vi "PhotonMultiTargetPNPResult_unpack.vi"(9 "StartByte":i32, 11 "RawData":u8[](array[numeric])) -> (1 "NextByte":i32, 3 "MultiTargetPNP_Result":T1={"PhotonPNPResult"={"IsPresent"=FALSE, "bestReprojErr"=0.0, "altReprojErr"=0.0, "ambiguity"=0.0, "Best"={"TRANSLATION3D"={"X"=0.0, "Y"=0.0, "Z"=0.0}, "ROTATION3D"={"Q_quaternion"={"R"=1.0, "V"=[0.0, 0.0, 0.0]}}, "XF"=FALSE}, "Alt"={"TRANSLATION3D"={"X"=0.0, "Y"=0.0, "Z"=0.0}, "ROTATION3D"={"Q_quaternion"={"R"=1.0, "V"=[0.0, 0.0, 0.0]}}, "XF"=FALSE}}, "FiducialIDsUsed"=[]} {"PhotonPNPResult"."Alt"."TRANSLATION3D"."Z" format="%14.3f"; "PhotonPNPResult"."Alt"."TRANSLATION3D"."Y" format="%14.3f"; "PhotonPNPResult"."Alt"."TRANSLATION3D"."X" format="%14.3f"; "PhotonPNPResult"."Best"."TRANSLATION3D"."Z" format="%14.3f"; "PhotonPNPResult"."Best"."TRANSLATION3D"."Y" format="%14.3f"; "PhotonPNPResult"."Best"."TRANSLATION3D"."X" format="%14.3f"})   [LabVIEW 2019, in "PhotonVisionLib.lvlib"]
doc: "Internal function to parse the data for each target returned by PhotonCamera_GetLatestResult.\n\nInputs:\n - RawData -- Byte array containing the data to parse.\n\nOutputs:\n - TrackedTarget -- Parsed TrackedTarget cluster."
uses:
  PhotonVisionLib.lvlib
  TypeDef/PhotonMultiTargetPNPResultType.ctl
  TypeDef/PhotonPNPResultType.ctl
  <vilib>/Rock Robotics/WPI/ThirdParty/JAS_Junk/TrajLib/TypeDef/TRANSFORM3D.ctl
  <vilib>/Rock Robotics/WPI/ThirdParty/JAS_Junk/TrajLib/TypeDef/TRANSLATION3D.ctl
  <vilib>/Rock Robotics/WPI/ThirdParty/JAS_Junk/TrajLib/TypeDef/ROTATION3D.ctl
  <vilib>/Rock Robotics/WPI/ThirdParty/JAS_Junk/TrajLib/TypeDef/QUATERNION.ctl
  Packet_decode_Boolean.vi
  PhotonPNPResult_New_Empty.vi
  Packet_decode_Transform3d.vi
  Packet_decode_Flt64.vi
  PhotonPNPResult_New.vi
  <vilib>/Rock Robotics/WPI/ThirdParty/JAS_Junk/TrajLib/VI/Transform3d_Create_Trans3dRot3d.vi
  <vilib>/Rock Robotics/WPI/ThirdParty/JAS_Junk/TrajLib/VI/Translation3d_Create.vi
  <vilib>/Rock Robotics/WPI/ThirdParty/JAS_Junk/TrajLib/VI/Rotation3d_Create_Quaternion.vi
  <vilib>/Rock Robotics/WPI/ThirdParty/JAS_Junk/TrajLib/VI/Quaternion_New.vi
  <vilib>/Rock Robotics/WPI/ThirdParty/JAS_Junk/TrajLib/VI/Quaternion_Normalize.vi
  <vilib>/Rock Robotics/WPI/ThirdParty/JAS_Junk/TrajLib/VI/Quaternion_New_Default.vi
  <vilib>/Rock Robotics/WPI/ThirdParty/JAS_Junk/TrajLib/Trajectory_Library.lvlib
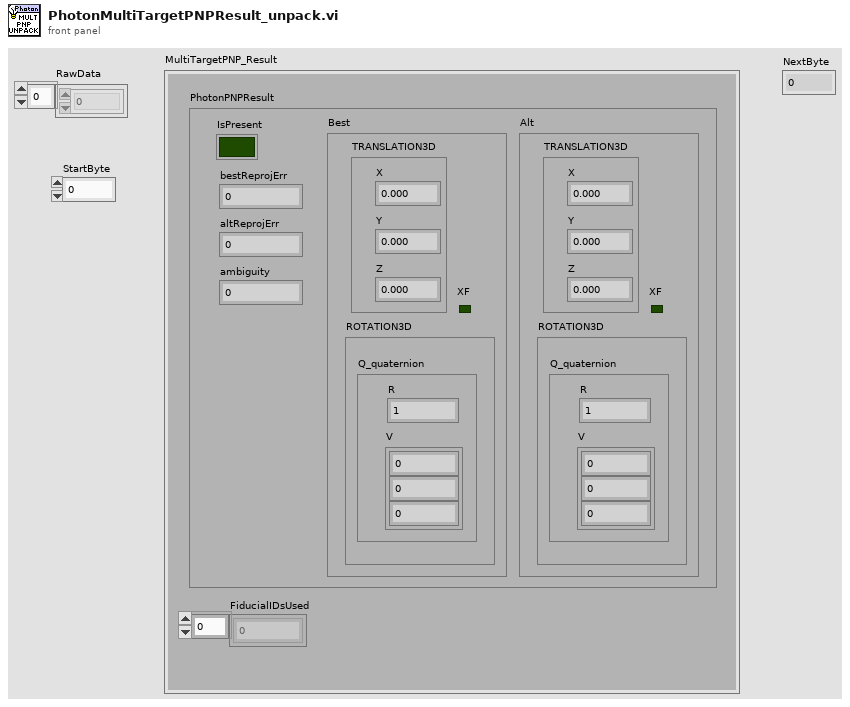
[diagram p1: front panel]
types:
  T1 = typedef "PhotonVisionLib.lvlib/PhotonMultiTargetPNPResultType.ctl" = cluster{"PhotonPNPResult":T2, "FiducialIDsUsed":i16[]}
  T2 = typedef "PhotonVisionLib.lvlib/PhotonPNPResultType.ctl" = cluster{"IsPresent":bool, "bestReprojErr":dbl, "altReprojErr":dbl, "ambiguity":dbl, "Best":T3, "Alt":T3}
  T3 = typedef "Trajectory_Library.lvlib/TRANSFORM3D.ctl" = cluster{"TRANSLATION3D":T4, "ROTATION3D":T5, "XF":bool}
  T4 = typedef "Trajectory_Library.lvlib/TRANSLATION3D.ctl" = cluster{"X":dbl, "Y":dbl, "Z":dbl}
  T5 = typedef "Trajectory_Library.lvlib/ROTATION3D.ctl" = cluster{"Q_quaternion":T6}
  T6 = typedef "Trajectory_Library.lvlib/QUATERNION.ctl" = cluster{"R":dbl, "V":dbl[]}
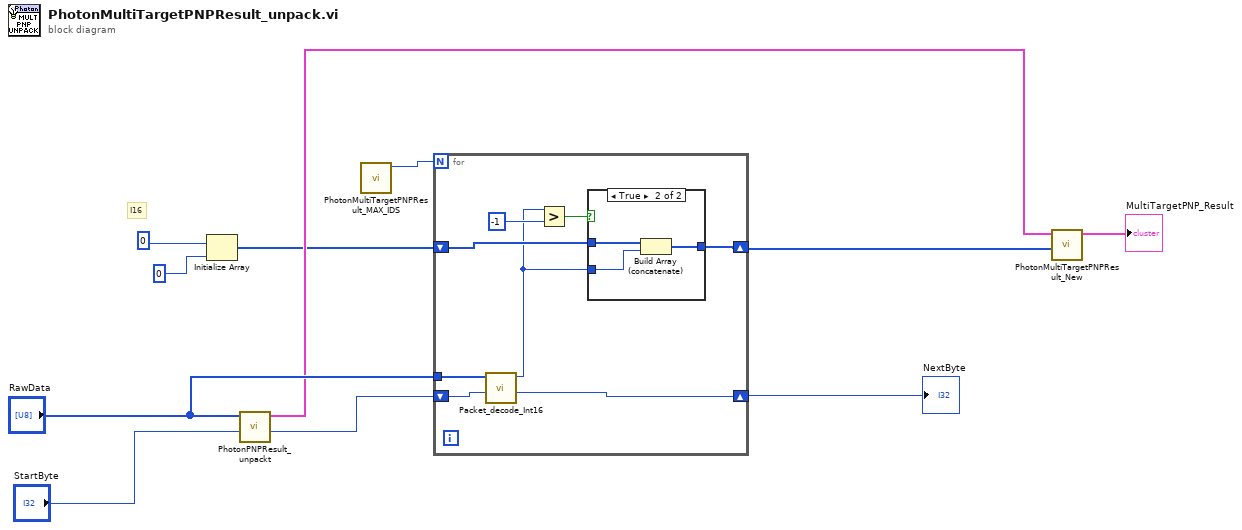
[diagram p0: block diagram]
diagram:
  # "I16"
  n1 = Initialize Array(i16 0, 0 ("dimension size")) -> (w2:i16[])
  n2 = call "PhotonPNPResult_unpackt.vi"("StartByte"="StartByte", "RawData"="RawData") -> ("NextByte"=w7:i32, "PNP_Result"=w6:T2)  [unwired: 8 in]
  n3 = call "PhotonMultiTargetPNPResult_MAX_IDS.vi"() -> ("MAX_IDS"=w9:i32)  [unwired: 11 in]
  n4 = for {
    N: w9 -> [_]
    tunnel: "RawData" -> [w19]
    shift-right: [w17] -> w5
    shift-left: w7 -> [w18]
    shift-right: [w12] -> w1
    shift-left: w2 -> [w14]
    n5 = call "Packet_decode_Int16.vi"("StartByte"=w18, "RawData"=w19) -> ("NextByte"=w17:i32, "Int16_Value"=w13:i16)  [unwired: 8 in]
    n6 = Greater?(x=w13, y=i16 -1) -> (0:w15:bool)
    n7 = case shown="True" w15 {
      tunnel: w14 -> [w20 w23]
      tunnel: w13 -> [_ w22]
      tunnel: [w20 w21] -> w12
      frame False {
      }
      frame True {
        n8 = Build Array (concatenate)(w23, w22) -> (w21:i16[])
      }
    }
  }
  "NextByte" <- w5
  n9 = call "PhotonMultiTargetPNPResult_New.vi"("FiducialIDsUsed"=w1, "PhotonPNPResult"=w6) -> ("MultiTargetPNPResult"=→"MultiTargetPNP_Result":T1)  [unwired: 9 in]
